vi "Write CurrentPCFG.vi"(8 "Error In":errorcluster, 10 "File Path":path) -> (0 "Error Out":errorcluster)   [LabVIEW 2014, in "Standard Editor.lvlib" / "DCAF INI.lvlib"]
doc: "Writes Path input to CurrentPCFG INI token."
uses:
  DCAF INI.lvlib
  <vilib>/Utility/config.llb/Write Key (Path).vi
  <vilib>/Utility/config.llb/NI_LVConfig.lvlib
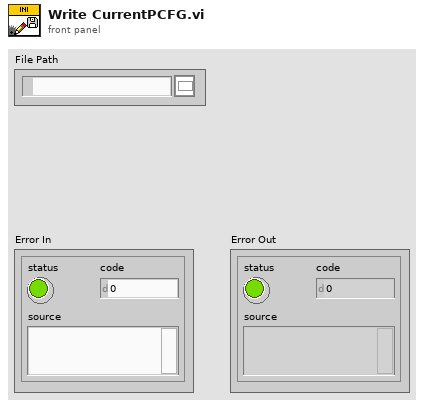
[diagram p1: front panel]
types:
  T1 = typedef "NI_LVConfig.lvlib/Config Data RefNum.ctl" = refnum<k1>
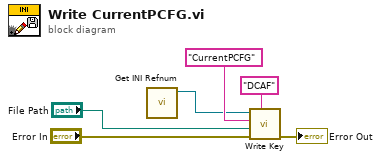
[diagram p0: block diagram]
diagram:
  n1 = call "Get INI Refnum.vi"() -> ("INI Refnum Out"=w1:T1)  [unwired: 11 in]
  n2 = call-poly <vilib>:"Write Key.vi"("section"="DCAF", "error in (no error)"="Error In", "value"="File Path", "key"="CurrentPCFG", "refnum"=w1) -> ("error out"=→"Error Out":errorcluster)  [unwired: 4 in, 2 out]
